vi "Rot_pot_voltage_to_degree.vi"(1 "RotaryPot (Voltage)":dbl) -> (0 "RotaryPot (degree)":dbl)   [LabVIEW 2019]
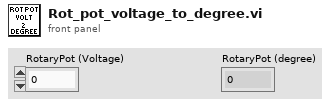
[diagram p1: front panel]
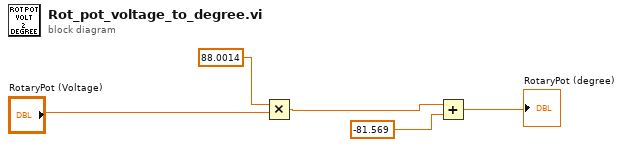
[diagram p0: block diagram]
diagram:
  n1 = Multiply(x=88.0014, y="RotaryPot (Voltage)") -> (x*y=w5:dbl)
  n2 = Add(x=w5, y=-81.569) -> (x+y=→"RotaryPot (degree)":dbl)
